vi "JKI Python Bridge - Example.vi"() -> ()   [LabVIEW 2020]
uses:
  Server/Type Definitions/Python Method.ctl
  303f235d-b2b7-4d3d-96b2-58cf21ef0f33.vi
  d3cf6f6b-a4fd-42ef-8031-03215f8826f1.vi
  6580c6d9-ce86-4ac9-8159-b199db024025.vi
  3fdd420e-69a3-492a-b553-cd64ded51656.vi
  861de6d6-96a5-4a62-93db-31956d419962.vi
  Server/Register for Events (Single PyObject).vi
  Call/Send Return Value.vi
  Python Data Tools/source/Python String to LabVIEW Data.vi
  Python Data Tools/source/Python String to LabVIEW Data/Python String to LabVIEW Data (Variant).vi
  Server/Server.lvclass
  Call/Call.lvclass
panel:
  in  "Show LabVIEW.py in Explorer":bool
  in  "Open Python":bool
  in  "Exit":bool
  out "Client Connected":bool
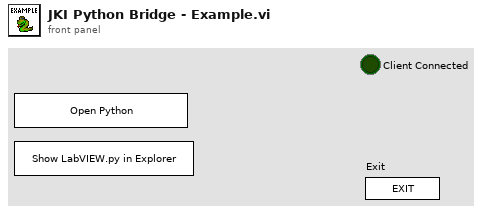
[diagram p1: front panel]
types:
  T1 = typedef "jki_python_bridge.lvlib/Server.lvclass/Python Method.ctl" = cluster{"Name":string, "Arguments":string[], "Documentation":string}
  T2 = typedef "jki_python_bridge.lvlib/Server.lvclass/Python Method Call - Event Registration.ctl" = refnum<event-registration>
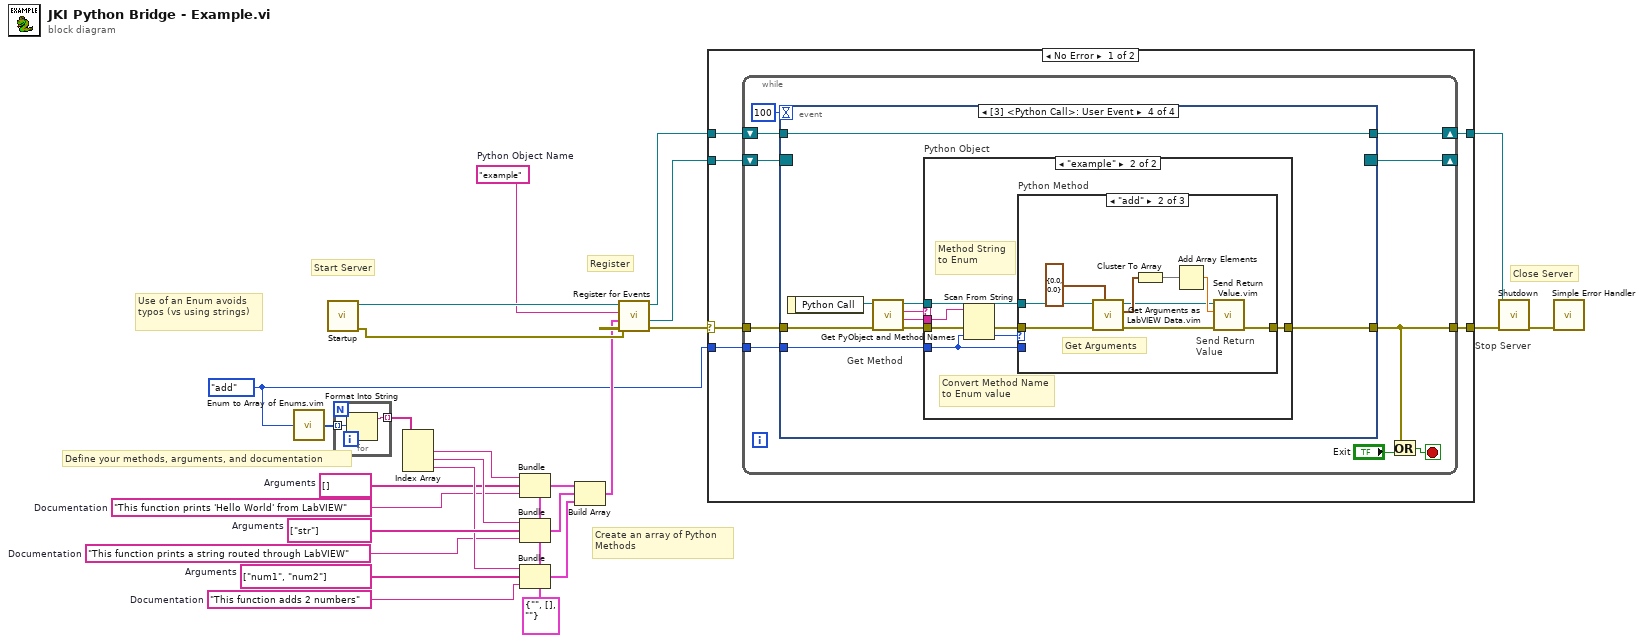
[diagram p0: block diagram]
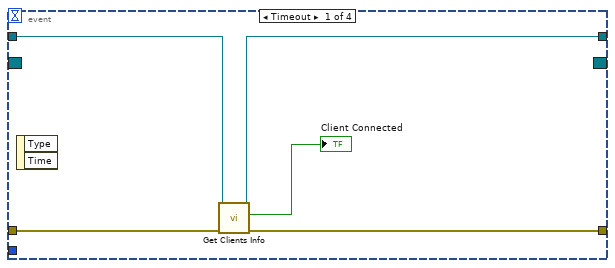
[diagram p2: hidden frame]
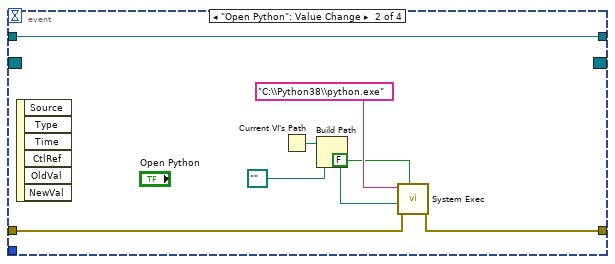
[diagram p3: hidden frame]
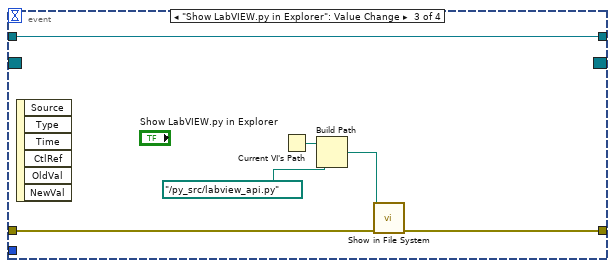
[diagram p4: hidden frame]
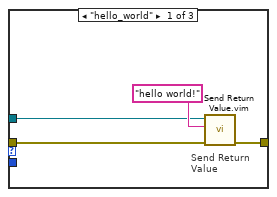
[diagram p6: hidden frame]
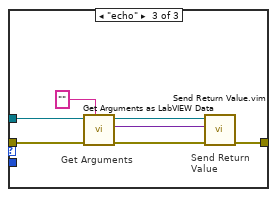
[diagram p7: hidden frame]
diagram:
  w5 = string[] []  # Arguments
  w6 = T1 {"Name"="", "Arguments"=[], "Documentation"=""} ("Method")
  w7 = "This function adds 2 numbers"  # Documentation
  w8 = "This function prints a string routed through LabVIEW"  # Documentation
  w9 = "This function prints 'Hello World' from LabVIEW"  # Documentation
  w15 = string[] ["num1", "num2"]  # Arguments
  w16 = string[] ["str"]  # Arguments
  w3 = enum16{"hello_world", "echo", "add"}."add"
  w22 = "example"  # Python Object Name
  # "Close Server"
  # "Create an array of Python \nMethods"
  # "Define your methods, arguments, and documentation"
  # "Register"
  # "Start Server"
  # "Use of an Enum avoids typos (vs using strings)"
  n1 = call "Enum to Array of Enums.vim"("enum"=w3) -> ("array of enums"=w2:enum16{"hello_world", "echo", "add"}[])
  n2 = call "Startup.vi"() -> ("error out"=w24:errorcluster, "JKI_Python_Server out"=w23:refnum<class "Server.lvclass">)  [unwired: 10 in]
  n3 = for {
    tunnel: w2 -> [w28] mode=indexing
    tunnel: [w27] -> w1 mode=indexing
    n4 = Format Into String(w28) -> (resulting string=w27:string)  [unwired: 3 in, 1 out]
  }
  n5 = Index Array(array=w1) -> (element #1=w18:string, element #2=w17:string, element #3=w14:string)  [unwired: 3 in]
  n6 = Bundle(cluster=w6, "Name"=w18, "Arguments"=w5, "Documentation"=w9) -> (w13:T1)
  n7 = Bundle(cluster=w6, "Name"=w17, "Arguments"=w16, "Documentation"=w8) -> (w12:T1)
  n8 = Bundle(cluster=w6, "Name"=w14, "Arguments"=w15, "Documentation"=w7) -> (w11:T1)
  n9 = Build Array(w13, w12, w11) -> (w10:T1[])
  n10 = call-poly "Register for Events.vi"("error in (no error)"=w24, "Functions"=w10, "PyObject Name"=w22, "JKI_Python_Server in"=w23) -> ("error out"=w21:errorcluster, "Python"=w20:T2, "JKI_Python_Server out"=w19:refnum<class "Server.lvclass">)  [unwired: 5 in]
  n11 = case shown="No Error" w21 {
    selector: w21 -> [w31 w101]
    tunnel: [w34 w102] -> w26
    tunnel: [w33 w101] -> w25
    tunnel: w3 -> [w32 _]
    tunnel: w20 -> [w30 _]
    tunnel: w19 -> [w29 w102]
    frame No Error {
      # "Stop Server"
      n12 = while {
        shift-right: [w40] -> w34
        shift-left: w29 -> [w41]
        shift-right: [w39] -> _
        shift-left: w30 -> [w44]
        tunnel: w32 -> [w37]
        tunnel: w31 -> [w43]
        tunnel: [w35] -> w33
        stop <- w36 stop-if-true
        n13 = event shown="[3] <Python Call>: User Event" {
          selector: w44 -> [_ _ _ _]
          dyn-events: [_ _ _ _] -> w39
          timeout: 100 -> [_ _ _ _]
          tunnel: [w47 w51 w58 w66] -> w35
          tunnel: w43 -> [w48 w52 w59 w70]
          tunnel: w41 -> [w49 w57 w63 w72]
          tunnel: [w45 w57 w63 w72] -> w40
          tunnel: w37 -> [_ _ _ w67]
          event Timeout {
            n14 = event-data() -> ()  [unwired: 1 in, 2 out]
            n15 = call "Get Clients Info.vi"("error in (no error)"=w48, "JKI_Python_Server in"=w49) -> ("error out"=w47:errorcluster, "Client Connected"=→"Client Connected":bool, "JKI_Python_Server out"=w45:refnum<class "Server.lvclass">)  [unwired: 5 in, 2 out]
          }
          event "Open Python": Value Change {
            n16 = event-data() -> ()  [unwired: 1 in, 6 out]
            n17 = Current VI's Path() -> (path=w56:path)
            n18 = Build Path(base path=w56, name or relative path=path "..") -> (appended path=w53:path)
            n19 = call <vilib>:"System Exec.vi"("wait until completion? (T)"=FALSE, "error in (no error)"=w52, "working directory"=w53, "command line"="C:\\Python38\\python.exe") -> ("error out"=w51:errorcluster)  [unwired: 4 in, 3 out]
          }
          event "Show LabVIEW.py in Explorer": Value Change {
            n20 = event-data() -> ()  [unwired: 1 in, 6 out]
            n21 = Current VI's Path() -> (path=w62:path)
            n22 = Build Path(base path=w62, name or relative path=path "../py_src/labview_api.py") -> (appended path=w60:path)
            n23 = call <vilib>:"Show in File System.vi"("error in (no error)"=w59, "file or directory path"=w60) -> ("error out"=w58:errorcluster)  [unwired: 9 in]
          }
          event User Event {
            # "Get Method"
            n24 = event-data() -> ("Python Call"=w71:refnum<class "Call.lvclass">)  [unwired: 1 in]
            n25 = call "Get PyObject and Method Names.vi"("error in (no error)"=w70, "Call in"=w71) -> ("error out"=w69:errorcluster, "Method Name"=w65:string, "PyObject Name"=w64:string, "Call out"=w68:refnum<class "Call.lvclass">)  [unwired: 5 in, 1 out]
            n26 = case "Python Object" shown="\"example\"" w64 {
              tunnel: w69 -> [w73 w75]
              tunnel: w68 -> [_ w79]
              tunnel: w67 -> [_ w78]
              tunnel: [w73 w77] -> w66
              tunnel: w65 -> [_ w76]
              frame Default {
              }
              frame "example" {
                # "Convert Method Name to Enum value"
                # "Method String to Enum"
                n27 = Scan From String(input string=w76, error in=w75, default 1=w78) -> (error out=w74:errorcluster, output 1=w80:enum16{"hello_world", "echo", "add"})  [unwired: 2 in, 2 out]
                n28 = case "Python Method" shown="\"add\"" w80 {
                  tunnel: w74 -> [w84 w92 w99]
                  tunnel: [w83 w86 w96] -> w77
                  tunnel: w79 -> [w81 w93 w100]
                  tunnel: w78 -> [_ _ _]
                  frame "hello_world" {
                    # "Send Return\nValue"
                    n29 = call "Send Return Value.vim"("error in (no error)"=w84, "Return Value"="hello world!" ("Arguments"), "Response in"=w81) -> ("error out"=w83:errorcluster)  [unwired: 8 in]
                  }
                  frame "add" {
                    # "Send Return\nValue"
                    # "Get Arguments"
                    n30 = call "Get Arguments as LabVIEW Data.vim"("type"=cluster{dbl, dbl} {0.0, 0.0}, "error in (no error)"=w92, "Call in"=w93) -> ("error out"=w87:errorcluster, "LabVIEW Data"=w89:cluster{dbl, dbl}, "Call out"=w85:refnum<class "Call.lvclass">)  [unwired: 6 in]
                    n31 = Cluster To Array(cluster=w89) -> (array=w90:dbl[])
                    n32 = Add Array Elements(numeric array=w90) -> (sum=w88:dbl)
                    n33 = call "Send Return Value.vim"("error in (no error)"=w87, "Return Value"=w88, "Response in"=w85) -> ("error out"=w86:errorcluster)  [unwired: 8 in]
                  }
                  frame "echo" {
                    # "Send Return\nValue"
                    # "Get Arguments"
                    n34 = call "Get Arguments as LabVIEW Data.vi"("type"="", "error in (no error)"=w99, "Call in"=w100) -> ("error out"=w97:errorcluster, "LabVIEW Data"=w95:variant, "Call out"=w94:refnum<class "Call.lvclass">)  [unwired: 6 in]
                    n35 = call "Send Return Value.vim"("error in (no error)"=w97, "Return Value"=w95, "Response in"=w94) -> ("error out"=w96:errorcluster)  [unwired: 8 in]
                  }
                }
              }
            }
          }
        }
        n36 = Or(x=w35, y="Exit") -> (x .or. y?=w36:bool)
      }
    }
    frame Error {
    }
  }
  n37 = call "Shutdown.vi"("error in (no error)"=w25, "JKI_Python_Server in"=w26) -> ("error out"=w4:errorcluster)  [unwired: 9 in]
  n38 = call <vilib>:"Simple Error Handler.vi"("error in (no error)"=w4) -> ()  [unwired: 4 in, 5 out]
